vi "get_layer_state.vi"(8 "error in (no error)":errorcluster, 10 "Layer":u8=1, 11 "VISA resource name":refnum<visa-resource-name>) -> (0 "error out":errorcluster, 2 "formatted response":string, 3 "VISA resource name out":refnum<visa-resource-name>)   [LabVIEW 2018]
doc: "Query structure, compatibility, and range version numbers."
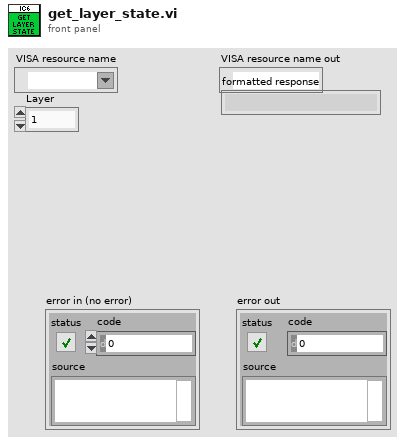
[diagram p1: front panel]
types:
  T1 = enum16{"Source", "General", "Input name", "Process name", "Logic", "Material", "Material name", "Output name", "Process", "Sensor", "Output type", "User message", "Layer", ""}
  T2 = enum16{"Hello", "Query", "Remote action", "Status", "Update"}
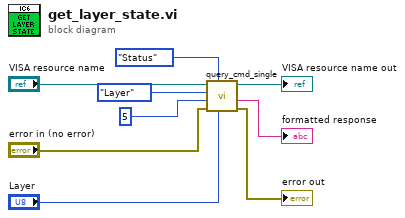
[diagram p0: block diagram]
diagram:
  n1 = call "query_cmd_single.vi"("Parameter"="Layer", "Command group"=T2."Status", "error in (no error)"="error in (no error)", "Command ID"=u8 5, "Command subgroup"=T1."Layer", "VISA resource name"="VISA resource name") -> ("error out"=→"error out":errorcluster, "formatted response"=→"formatted response":string, "VISA resource name out"=→"VISA resource name out":refnum<visa-resource-name>)  [unwired: 1 in, 2 out]
